vi "FTDI_MPSSE_Close.vi"(8 "error in (no error)":errorcluster, 11 "Handler":u32) -> (0 "error out":errorcluster)   [LabVIEW 2018]
uses:
  dll/libMPSSE.dll
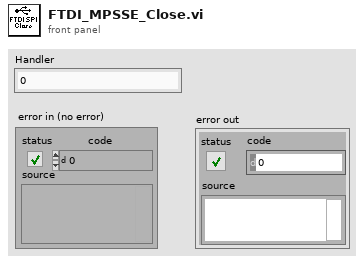
[diagram p1: front panel]
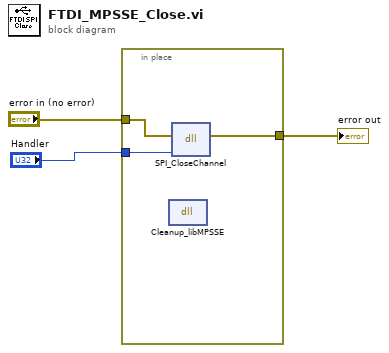
[diagram p0: block diagram]
diagram:
  n1 = in-place {
    in-place-border: "error in (no error)" -> [w6]
    in-place-border: [w5] -> w2
    in-place-border: "Handler" -> [w4]
    n2 = dll-call lib="D:/LABVIEW/Examples - 32bit/FTDI/libMPSSE-SPI-LabVIEW-master SNA - 01/dll/libMPSSE.dll" fn="Cleanup_libMPSSE"() -> ()  [unwired: 4 in, 2 out]
    n3 = dll-call lib="D:/LABVIEW/Examples - 32bit/FTDI/libMPSSE-SPI-LabVIEW-master SNA - 01/dll/libMPSSE.dll" fn="SPI_CloseChannel"(error in=w6, "handle"=w4) -> (error out=w5:errorcluster)  [unwired: 4 in, 1 out]
  }
  "error out" <- w2
